vi "Main Box Dome Control.vi"() -> ()   [LabVIEW 2019]
uses:
  RT Controls/Top Process Commands.ctl
  RT Controls/Top Command Events.ctl
  RT Controls/Main Process Commands.ctl
  RT Controls/Main Command Events.ctl
  <vilib>/FPGAPlugInAG/cRIO-9042/niLvFpga_Open_cRIO-9042.vi
  <vilib>/rvi/interface/common/dynamic/niFpgaDynamicAddResources.vi
  <vilib>/FPGAPlugInAG/Dynamic/niLvFpga_Run_Dynamic.vi
  <vilib>/Utility/error.llb/Error Cluster From Error Code.vi
  <vilib>/rvi/errors/niLvFpgaAdjustHostInterfaceError.vi
  <vilib>/FPGAPlugInAG/Dynamic/niLvFpga_Close_Dynamic.vi
  <vilib>/rvi/interface/nirviOpenFPGA/nirviOpenFPGA.xnode
  FPGA Bitfiles/auxtelmaindomeco_FPGATarget2_fpga_OJwirRnewPE.lvbitx
  <vilib>/rvi/interface/nirviMethod/nirviMethod.xnode
  <vilib>/rvi/interface/nirviReadWriteControl/nirviReadWriteControl.xnode
  <vilib>/rvi/interface/nirviCloseFPGA/nirviCloseFPGA.xnode
  NiFpgaLv.dll
  <vilib>/rvi/interface/Simulation/niFpgaSimulationCallBeginRW.vi
  <vilib>/NI_Real-Time Target Support.lvlib
panel:
  out "led":bool
  out "main queue":refnum<queue>
  out "top queue":refnum<queue>
  out "FPGA Error":errorcluster
  in  "stop":bool
  # "Main Box\nv03.0"
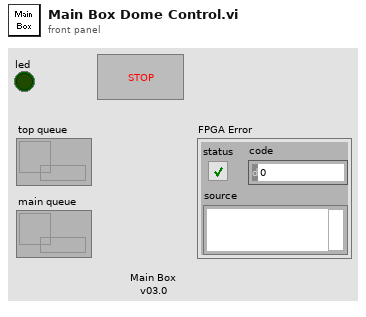
[diagram p1: front panel]
types:
  T1 = typedef "Top Process Commands.ctl" = cluster{"Command":T2, "Value":variant}
  T2 = typedef "Top Command Events.ctl" = enum16{"Idle", "FullStop", "ReadConfig", "WriteConfig", "OpenUpper", "CloseUpper", "OpenLower", "CloseLower", "SetWatchdogInt", "EnRainShutDn", "DisRainShutDn", "SetDoorMoveTO", "EnAutoShutDn", "DisAutoShutDn", "SetRevDelay", "SetRainDelay", "SyncClose", "SyncOpen"}
  T3 = typedef "Main Process Commands.ctl" = cluster{"Commands":T4, "Value":variant}
  T4 = typedef "Main Command Events.ctl" = enum16{"Idle", "FullStop", "MainReadConfig", "MainWriteConfig", "OpenUpper", "CloseUpper", "OpenLower", "CloseLower", "SetWatchdogInt", "EnCloudShutDn", "DisCloudShutDn", "SetRainDelay", "EnAutoShutDn", "DisAutoShutDn", "SetRevDelay", "RotToAz", "RotLeft", "RotRight", "RotToHome", "DefineHomePos", "SetHSThres", "SetEncCounts", "SyncClose", "SyncOpen", "SetAZTimLim", "SetAZTol", "AZEncPositive", "AZEncNegative", "RotToCenter"}
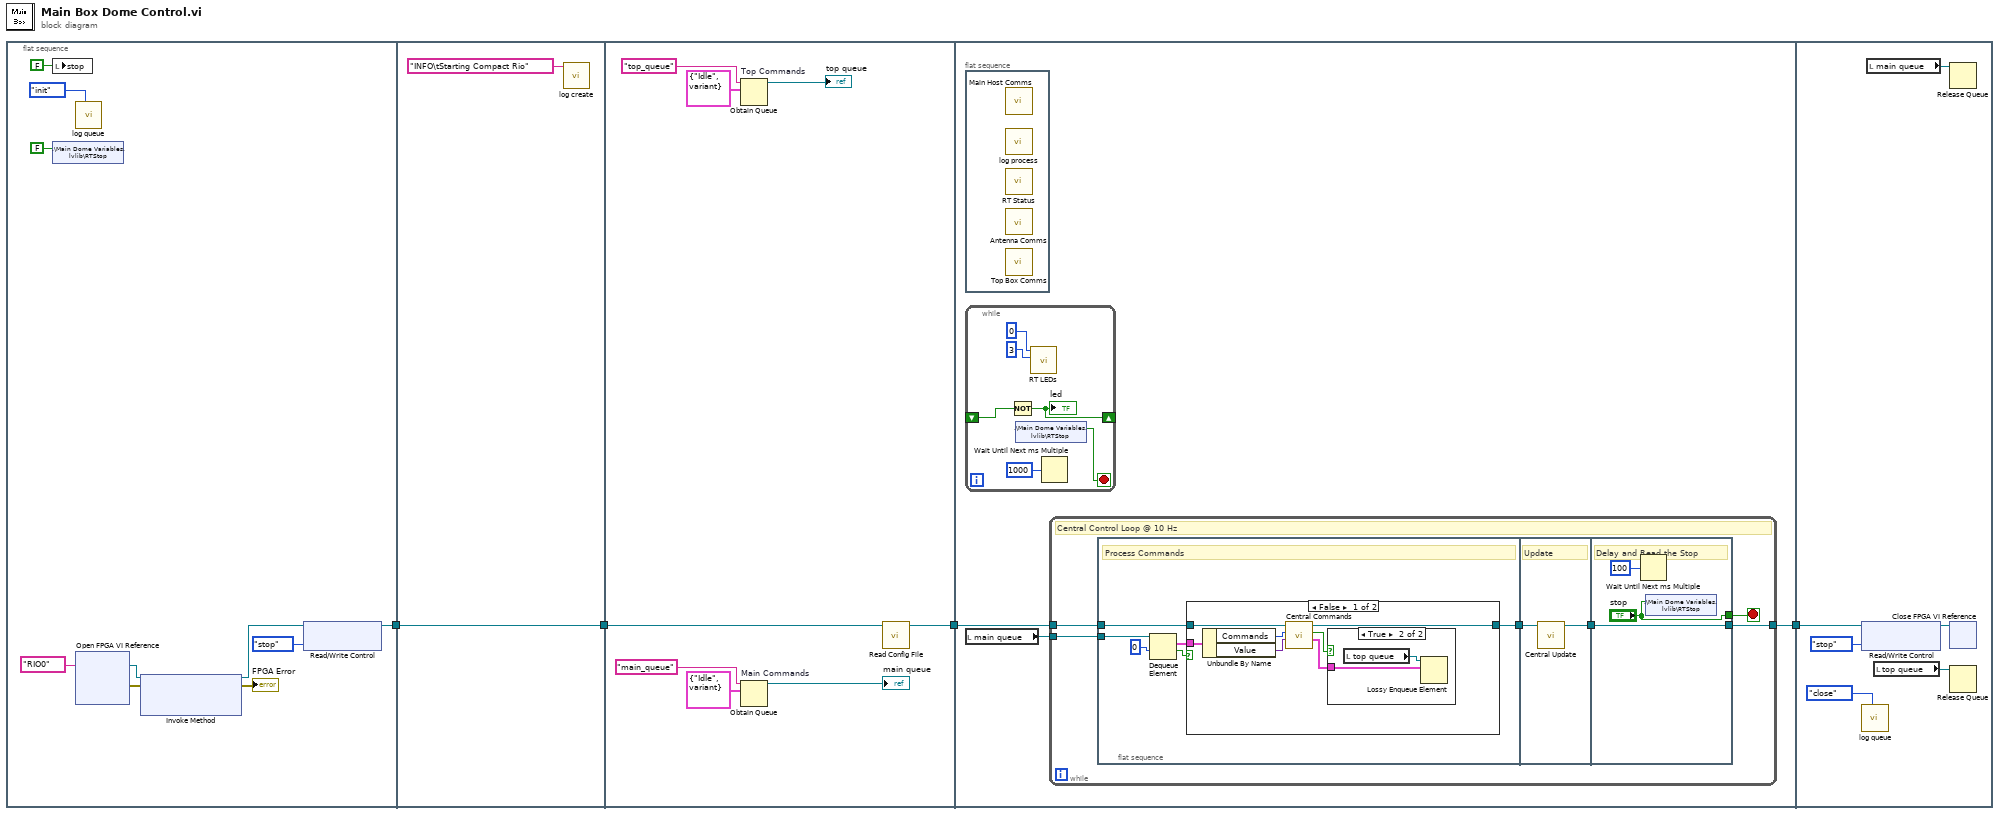
[diagram p0: block diagram]
diagram:
  n1 = flat-sequence {
    tunnel: [w8] -> w2
    tunnel: w2 -> [w16]
    tunnel: [w16] -> w1
    tunnel: w1 -> [w20]
    tunnel: [w19] -> w4
    tunnel: w4 -> [w27]
    tunnel: [w26] -> w3
    tunnel: w3 -> [w66]
    frame #0 {
      n2 = local write "stop"(FALSE ("stop")) -> ()
      n3 = shared-variable ".\\Main Dome Variables.lvlib\\RTStop"(FALSE ("RTStop")) -> ()  [unwired: 1 in, 1 out]
      n4 = call "log queue.vi"("action (get)"=enum16{"init", "get", "close"}."init") -> ()  [unwired: 10 in, 1 out]
      n5 = xnode "Open FPGA VI Reference"("resource name"=tag "RIO0") -> ("FPGA VI Reference Out"=w12:refnum<k20>, "error out"=w11:errorcluster)  [unwired: 1 in]
      n6 = xnode "Invoke Method"("FPGA VI Reference In"=w12, "error in"=w11) -> ("FPGA VI Reference Out"=w9:refnum<k20>, "error out"=→"FPGA Error":errorcluster)  [unwired: 1 in]
      n7 = xnode "Read/Write Control"("FPGA VI Reference In"=w9, "mode request"=enum16{"stop", "home", "position", "center"}."stop") -> ("FPGA VI Reference Out"=w8:refnum<k20>)  [unwired: 1 in, 1 out]
    }
    frame #1 {
      n8 = call "log create.vi"("message"="INFO\tStarting Compact Rio") -> ()  [unwired: 11 in]
    }
    frame #2 {
      n9 = Obtain Queue "Top Commands"(name (unnamed)="top_queue", element data type=T1 {"Command"=enum."Idle", "Value"=variant} ("ProcessEvents")) -> (queue out=→"top queue":refnum<queue>)  [unwired: 3 in, 2 out]
      n10 = Obtain Queue "Main Commands"(name (unnamed)="main_queue", element data type=T3 {"Commands"=enum."Idle", "Value"=variant} ("ProcessEvents")) -> (queue out=→"main queue":refnum<queue>)  [unwired: 3 in, 2 out]
      n11 = call "Read Config File.vi"("ref in"=w20) -> ("ref out"=w19:refnum<k20>)  [unwired: 10 in]
    }
    frame #3 {
      n12 = flat-sequence {
        frame #0 {
          n13 = call "Main Host Comms.vi"() -> ()  [unwired: 12 in]
          n14 = call "log process.vi"() -> ()  [unwired: 12 in]
          n15 = call "RT Status.vi"() -> ()  [unwired: 12 in]
          n16 = call "Antenna Comms.vi"() -> ()  [unwired: 12 in]
          n17 = call "Top Box Comms.vi"() -> ()  [unwired: 12 in]
        }
      }
      n18 = while {
        shift-right: [w29] -> _
        shift-left: _ -> [w30]
        stop <- w28 stop-if-true
        n19 = Not(x=w30) -> (.not. x?=w29:bool)
        "led" <- w29
        n20 = shared-variable ".\\Main Dome Variables.lvlib\\RTStop"() -> (w28:bool)  [unwired: 1 in, 1 out]
        n21 = call <vilib>:"RT LEDs.vi"("State"=3, "LED Num"=0) -> ()  [unwired: 4 in, 2 out]
        n22 = Wait Until Next ms Multiple(millisecond multiple=u32 1000) -> ()  [unwired: 1 out]
      }
      n23 = local read "main queue"() -> (w25:refnum<queue>)
      n24 = while {
        tunnel: w25 -> [w39]
        tunnel: w27 -> [w37]
        tunnel: [w36] -> w26
        stop <- w38 stop-if-true
        # "Central Control Loop @ 10 Hz"
        n25 = flat-sequence {
          tunnel: w39 -> [w44]
          tunnel: w37 -> [w41]
          tunnel: [w40] -> w35
          tunnel: w35 -> [w57]
          tunnel: [w56] -> w34
          tunnel: ["stop"] -> w38
          tunnel: [w58] -> w36
          tunnel: w34 -> [w58]
          frame #0 {
            # "Process Commands"
            n26 = Dequeue Element(queue=w44, timeout in ms (-1)=0) -> (element=w42:T3, timed out?=w43:bool)  [unwired: 1 in, 2 out]
            n27 = case shown="False" w43 {
              tunnel: w42 -> [w52 _]
              tunnel: w41 -> [w48 w55]
              tunnel: [w47 w55] -> w40
              frame False {
                n28 = Unbundle By Name(w52) -> ("Commands"=w50:T4, "Value"=w51:variant)
                n29 = call "Central Commands.vi"("Value"=w51, "Commands"=w50, "ref in"=w48) -> ("element"=w49:T1, "top enqueue?"=w46:bool, "ref out"=w47:refnum<k20>)  [unwired: 6 in]
                n30 = case shown="True" w46 {
                  tunnel: w49 -> [_ w54]
                  frame False {
                  }
                  frame True {
                    n31 = local read "top queue"() -> (w53:refnum<queue>)
                    n32 = Lossy Enqueue Element(queue=w53, element=w54) -> ()  [unwired: 1 in, 4 out]
                  }
                }
              }
              frame True {
                # "Timeout do nothing"
              }
            }
          }
          frame #1 {
            # "Update"
            n33 = call "Central Update.vi"("ref in"=w57) -> ("ref out"=w56:refnum<k20>)  [unwired: 10 in]
          }
          frame #2 {
            # "Delay and Read the Stop"
            n34 = Wait Until Next ms Multiple(millisecond multiple=u32 100) -> ()  [unwired: 1 out]
            n35 = shared-variable ".\\Main Dome Variables.lvlib\\RTStop"("stop") -> ()  [unwired: 1 in, 1 out]
          }
        }
      }
    }
    frame #4 {
      n36 = xnode "Read/Write Control"("FPGA VI Reference In"=w66, "mode request"=enum16{"stop", "home", "position", "center"}."stop") -> ("FPGA VI Reference Out"=w65:refnum<k20>)  [unwired: 1 in, 1 out]
      n37 = call "log queue.vi"("action (get)"=enum16{"init", "get", "close"}."close") -> ()  [unwired: 10 in, 1 out]
      n38 = local read "main queue"() -> (w64:refnum<queue>)
      n39 = local read "top queue"() -> (w63:refnum<queue>)
      n40 = Release Queue(queue=w64) -> ()  [unwired: 2 in, 3 out]
      n41 = xnode "Close FPGA VI Reference"("FPGA VI Reference In"=w65) -> ()  [unwired: 1 in, 1 out]
      n42 = Release Queue(queue=w63) -> ()  [unwired: 2 in, 3 out]
    }
  }
